vi "Config Filter.vi"(0 "VISA resource name":refnum<visa-resource-name>, 5 "Filter (F: OFF)":bool, 7 "Line Filter (F: OFF)":bool, 11 "error in (no error)":errorcluster) -> (4 "VISA resource name out":refnum<visa-resource-name>, 15 "error out":errorcluster)   [LabVIEW 2016, in "Yokogawa WT200 Series.lvlib"]
doc: "This VI sends the filter on/off command to the WT200 Series."
uses:
  Yokogawa WT200 Series.lvlib
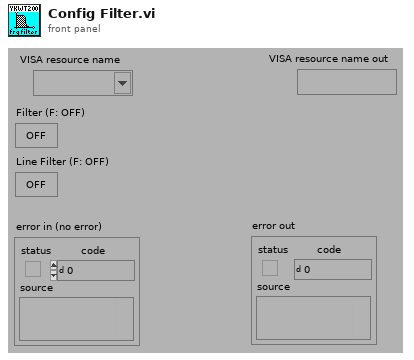
[diagram p1: front panel]
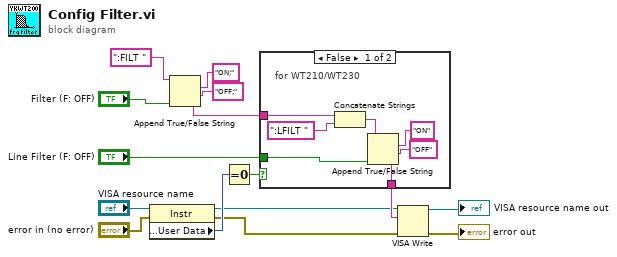
[diagram p0: block diagram]
diagram:
  n1 = property class="Instr"(reference="VISA resource name", error in="error in (no error)") -> (reference out=w2:refnum<visa-resource-name>, error out=w1:errorcluster, "General Settings:User Data"=w11:u32)
  n2 = Append True/False String(1:"Filter (F: OFF)", 2:"OFF;", 3:"ON;", 4:":FILT ") -> (0:w6:string)
  n3 = Equal To 0?(x=w11) -> (x = 0?=w10:bool)
  n4 = case shown="False" w10 {
    tunnel: "Line Filter (F: OFF)" -> [w20 _]
    tunnel: w6 -> [w17 w23]
    tunnel: [w16 w23] -> w3
    frame False {
      # "for WT210/WT230"
      n5 = Concatenate Strings(w17, ":LFILT ") -> (w18:string)
      n6 = Append True/False String(1:w20, 2:"OFF", 3:"ON", 4:w18) -> (0:w16:string)
    }
    frame True {
      # "for WT200"
    }
  }
  n7 = VISA Write(VISA resource name=w2, write buffer=w3, error in (no error)=w1) -> (VISA resource name out=→"VISA resource name out":refnum<visa-resource-name>, error out=→"error out":errorcluster)  [unwired: 1 out]
